vi "Random Data Generator.vi"(1 "Data Length":i32=10) -> (0 "Data":u8[](array[numeric]))   [LabVIEW 2014]
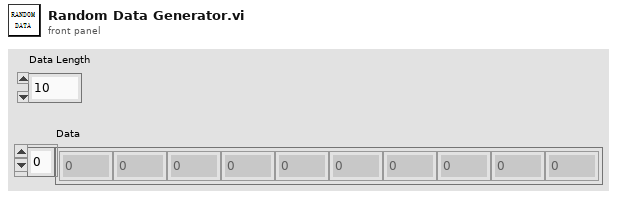
[diagram p1: front panel]
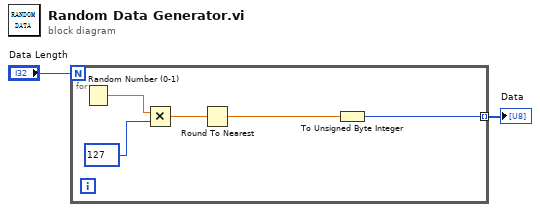
[diagram p0: block diagram]
diagram:
  n1 = for {
    N: "Data Length" -> [_]
    tunnel: [w3] -> w1 mode=indexing
    n2 = Random Number (0-1)() -> (number: 0 to 1=w7:dbl)
    n3 = Multiply(x=w7, y=127) -> (x*y=w5:dbl)
    n4 = Round To Nearest(number=w5) -> (nearest integer value=w4:dbl)
    n5 = To Unsigned Byte Integer(number=w4) -> (unsigned 8bit integer=w3:u8)
  }
  "Data" <- w1
